vi "4-probe measurement_new.vi"() -> ()   [LabVIEW 2011]
uses:
  <instrlib>/Keithley 24XX/Public/Data/Read (Multiple Points).vi
  <instrlib>/Keithley 2000/Public/Configure/Configure DC Volts.vi
  <instrlib>/Keithley 2000/Public/Configure/Configure AC Volts.vi
  <instrlib>/Keithley 2000/Public/Configure/Configure DC Current.vi
  <instrlib>/Keithley 2000/Public/Configure/Configure AC Current.vi
  <instrlib>/Keithley 2000/Public/Configure/Configure 2 Wire Resistance.vi
  <instrlib>/Keithley 2000/Public/Configure/Configure 4 Wire Resistance.vi
  <instrlib>/Keithley 24XX/Keithley 24XX.lvlib
  <instrlib>/Keithley 2000/Keithley 2000.lvlib
panel:
  out "XY Graph":cluster{"Y":dbl[], "Y":dbl[]}[](graph)
  in  "file path (use dialog)":path=path "C:/Documents and Settings/Professor/My Documents/LabVIEW Data/20130130/D2.txt"
  in  "Function (0: DC Volts)":u16(ring) items=["DC Volts", "AC Volts", "DC Current", "AC Current", "2-Wire Resistance", "4-Wire Resistance"]
  in  "2000 DMM":refnum<visa-resource-name>="GPIB::16"
  in  "Delay (0 s)":dbl
  in  "Number of Readings (10)":i32=10
  in  "Source Mode 2400  (0: Current)":u16(ring) items=["Voltage", "Current", "Resistance"]
  in  "Timeout (10000 ms)":i32=10000 format="%#.6g"
  in  "Number of Points (10)":u32=5
  in  "Maximum Amplitude (2)":dbl=2.0
  in  "Minimum Amplitude (1)":dbl=1.0
  in  "Compliance  Level (0.1)":dbl=0.1
  in  "Serial Configuration":T1={"Baud Rate"=9600, "Parity"=0, "Data Bits"=8, "Stop Bits"=10, "Flow Control"=0} {"Flow Control" items=["None", "XON/XOFF", "RTS/CTS", "XON/XOFF & RTS/CTS", "DTR/DSR", "XON/XOFF & DTR/DSR"]; "Stop Bits" items=["1.0"=10, "1.5"=15, "2.0"=20]; "Data Bits" items=["7"=7, "8"=8]; "Parity" items=["None", "Odd", "Even", "Mark", "Space"]; "Baud Rate" items=["300"=300, "600"=600, "1200"=1200, "2400"=2400, "4800"=4800, "9600"=9600, "19200"=19200]}
  in  "2400 Source Meter":refnum<visa-resource-name>
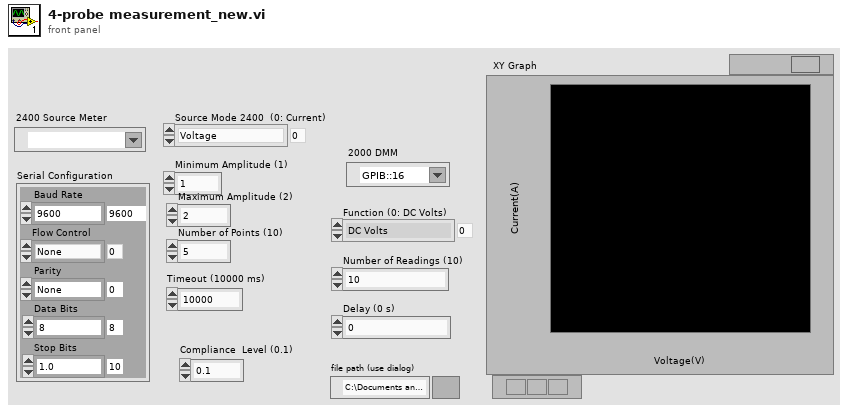
[diagram p1: front panel]
types:
  T1 = cluster{"Baud Rate":u32, "Parity":u16, "Data Bits":u16, "Stop Bits":u16, "Flow Control":u16}
  T2 = enum16{"open", "replace", "create", "open or create", "replace or create", "replace or create with confirmation"}
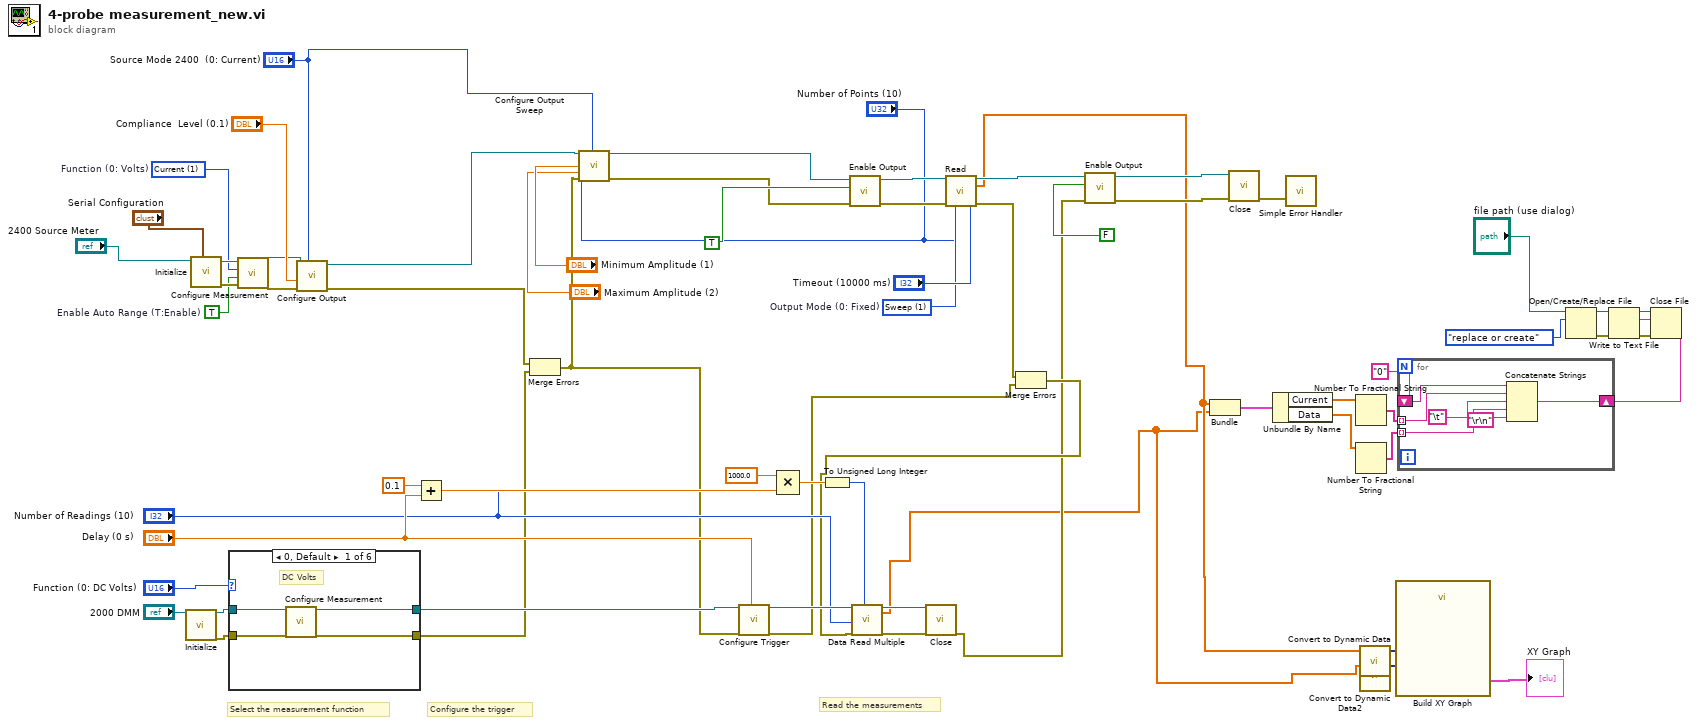
[diagram p0: block diagram]
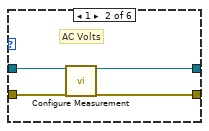
[diagram p2: hidden frame]
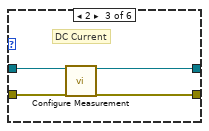
[diagram p3: hidden frame]
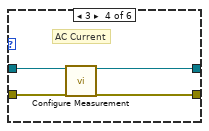
[diagram p4: hidden frame]
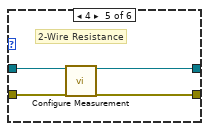
[diagram p5: hidden frame]
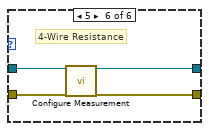
[diagram p6: hidden frame]
diagram:
  w47 = u16 1 items=["Fixed", "Sweep", "List"]  # Output Mode (0: Fixed)
  w62 = u16 1 items=["Volts", "Current", "Resistance"]  # Function (0: Volts)
  w61 = TRUE  # Enable Auto Range (T:Enable)
  # "Read the measurements"
  # "Configure the trigger"
  # "Select the measurement function"
  n1 = call <instrlib>:"Initialize.vi"("VISA resource name"="2000 DMM") -> ("VISA resource name out"=w27:refnum<visa-resource-name>, "error out"=w28:errorcluster)  [unwired: 17 in]
  n2 = call <instrlib>:"Initialize.vi"("Serial Configuration"="Serial Configuration", "VISA resource name"="2400 Source Meter") -> ("error out"=w63:errorcluster, "VISA resource name out"=w64:refnum<visa-resource-name>)  [unwired: 8 in]
  n3 = case shown="0, Default" "Function (0: DC Volts)" {
    tunnel: w28 -> [w70 w74 w78 w82 w86 w90]
    tunnel: w27 -> [w69 w73 w77 w81 w85 w89]
    tunnel: [w68 w72 w76 w80 w84 w88] -> w21
    tunnel: [w67 w71 w75 w79 w83 w87] -> w29
    frame 0, Default {
      # "DC Volts"
      n4 = call-poly <instrlib>:"Configure Measurement.vi"("VISA resource name"=w69, "error in (no error)"=w70) -> ("VISA resource name out"=w67:refnum<visa-resource-name>, "error out"=w68:errorcluster)  [unwired: 16 in]
    }
    frame 1 {
      # "AC Volts"
      n5 = call-poly <instrlib>:"Configure Measurement.vi"("VISA resource name"=w73, "error in (no error)"=w74) -> ("VISA resource name out"=w71:refnum<visa-resource-name>, "error out"=w72:errorcluster)  [unwired: 16 in]
    }
    frame 2 {
      # "DC Current"
      n6 = call-poly <instrlib>:"Configure Measurement.vi"("VISA resource name"=w77, "error in (no error)"=w78) -> ("VISA resource name out"=w75:refnum<visa-resource-name>, "error out"=w76:errorcluster)  [unwired: 16 in]
    }
    frame 3 {
      # "AC Current"
      n7 = call-poly <instrlib>:"Configure Measurement.vi"("VISA resource name"=w81, "error in (no error)"=w82) -> ("VISA resource name out"=w79:refnum<visa-resource-name>, "error out"=w80:errorcluster)  [unwired: 16 in]
    }
    frame 4 {
      # "2-Wire Resistance"
      n8 = call-poly <instrlib>:"Configure Measurement.vi"("VISA resource name"=w85, "error in (no error)"=w86) -> ("VISA resource name out"=w83:refnum<visa-resource-name>, "error out"=w84:errorcluster)  [unwired: 16 in]
    }
    frame 5 {
      # "4-Wire Resistance"
      n9 = call-poly <instrlib>:"Configure Measurement.vi"("VISA resource name"=w89, "error in (no error)"=w90) -> ("VISA resource name out"=w87:refnum<visa-resource-name>, "error out"=w88:errorcluster)  [unwired: 16 in]
    }
  }
  n10 = call <instrlib>:"Configure Measurement.vi"("error in (no error)"=w63, "Enable Auto Range (T:Enable)"=w61, "Function (0: Volts)"=w62, "VISA resource name"=w64) -> ("error out"=w58:errorcluster, "VISA resource name out"=w59:refnum<visa-resource-name>)  [unwired: 6 in]
  n11 = call <instrlib>:"Configure Output.vi"("Source Mode  (0: Voltage)"="Source Mode 2400  (0: Current)", "error in (no error)"=w58, "Compliance  Level (0.1)"="Compliance  Level (0.1)", "VISA resource name"=w59) -> ("error out"=w20:errorcluster, "VISA resource name out"=w43:refnum<visa-resource-name>)  [unwired: 6 in]
  n12 = Add(x=0.1, y="Delay (0 s)") -> (x+y=w33:dbl)
  n13 = Merge Errors "Merge Errors"(w20, w21) -> (w19:errorcluster)
  n14 = call <instrlib>:"Configure Output Sweep.vi"("VISA resource name"=w43, "Source Mode  (0: Voltage)"="Source Mode 2400  (0: Current)", "Number of Points (5)"="Number of Points (10)", "Minimum Amplitude (1)"="Minimum Amplitude (1)", "Maximum Amplitude (2)"="Maximum Amplitude (2)", "error in (no error)"=w19) -> ("VISA resource name out"=w42:refnum<visa-resource-name>, "error out"=w22:errorcluster)  [unwired: 8 in]
  n15 = call <instrlib>:"Configure Trigger.vi"("VISA resource name"=w29, "error in (no error)"=w19, "Delay (0 s)"="Delay (0 s)") -> ("VISA resource name out"=w39:refnum<visa-resource-name>, "error out"=w25:errorcluster)  [unwired: 15 in]
  n16 = Compound Arithmetic op=MULTIPLY(1000.0 ("x"), w33, "Number of Readings (10)") -> (w31:dbl)
  n17 = To Unsigned Long Integer(number=w31) -> (unsigned 32bit integer=w35:u32)
  n18 = call <instrlib>:"Enable Output.vi"("error in (no error)"=w22, "Enable Output (T: Enable)"=TRUE, "VISA resource name"=w42) -> ("error out"=w49:errorcluster, "VISA resource name out"=w50:refnum<visa-resource-name>)  [unwired: 7 in]
  n19 = call-poly <instrlib>:"Read.vi"("VISA resource name"=w50, "Sample Count (1)"="Number of Points (10)", "Timeout (10000 ms)"="Timeout (10000 ms)", "error in (no error)"=w49, "Output Mode (0: Fixed)"=w47) -> ("VISA resource name out"=w46:refnum<visa-resource-name>, "Current"=w2:sgl[], "error out"=w26:errorcluster)  [unwired: 4 in, 4 out]
  n20 = Merge Errors "Merge Errors"(w26, w25) -> (w24:errorcluster)
  n21 = call <instrlib>:"Data Read Multiple.vi"("VISA resource name"=w39, "Number of Readings (100)"="Number of Readings (10)", "error in (no error)"=w24, "Timeout (25000 ms)"=w35) -> ("VISA resource name out"=w40:refnum<visa-resource-name>, "Data"=w1:dbl[], "error out"=w41:errorcluster)  [unwired: 11 in, 2 out]
  n22 = call <instrlib>:"Close.vi"("VISA resource name"=w40, "error in (no error)"=w41) -> ("error out"=w23:errorcluster)  [unwired: 17 in]
  n23 = call <instrlib>:"Enable Output.vi"("error in (no error)"=w23, "Enable Output (T: Enable)"=FALSE, "VISA resource name"=w46) -> ("error out"=w55:errorcluster, "VISA resource name out"=w56:refnum<visa-resource-name>)  [unwired: 7 in]
  n24 = Bundle "Bundle"("Current"=w2, "Data"=w1) -> (w9:cluster{"Current":sgl[], "Data":dbl[]})  [unwired: 1 out]
  n25 = call <instrlib>:"Close.vi"("error in (no error)"=w55, "VISA resource name"=w56) -> ("error out"=w57:errorcluster)  [unwired: 9 in]
  n26 = Unbundle By Name "Unbundle By Name"(w9) -> ("Current"=w11:sgl[], "Data"=w10:dbl[])
  n27 = call <vilib>:"Simple Error Handler.vi"("error in (no error)"=w57) -> ()  [unwired: 4 in, 5 out]
  n28 = Number To Fractional String(number=w11) -> (F-format string=w18:string[])  [unwired: 3 out]
  n29 = Number To Fractional String(number=w10) -> (F-format string=w17:string[])  [unwired: 3 out]
  n30 = call "Convert to Dynamic Data"("Array"=w2) -> ("Dynamic Data Type"=w4:dynamicdata)  [unwired: 3 in]
  n31 = call "Convert to Dynamic Data2"("Array"=w1) -> ("Dynamic Data Type"=w3:dynamicdata)  [unwired: 3 in]
  n32 = call "Build XY Graph"("Y Input"=w3, "X Input"=w4) -> ("XY Graph"=→"XY Graph":cluster{"Y":dbl[], "Y":dbl[]}[])  [unwired: 3 in, 6 out]
  n33 = for {
    tunnel: w18 -> [w96] mode=indexing
    tunnel: w17 -> [w94] mode=indexing
    shift-right: [w92] -> w8
    shift-left: "0" -> [w91]
    n34 = Concatenate Strings "Concatenate Strings"(w91, w96, "\t", w94, "\r\n") -> (w92:string)
  }
  n35 = Open/Create/Replace File(file path (use dialog)="file path (use dialog)", operation (0:open)=T2."replace or create") -> (refnum out=w12:refnum<file>, error out=w16:errorcluster)  [unwired: 1 in, 4 out]
  n36 = Write to Text File(file (use dialog)=w12, text=w8, error in=w16) -> (refnum out=w14:refnum<file>, error out=w15:errorcluster)  [unwired: 2 out]
  n37 = Close File(refnum=w14, error in=w15) -> ()  [unwired: 2 out]
